vi "Mini Bach random sampling_type2_sub.vi"(0 "Mini Bach No.":i32, 1 "MNIST Input":i32[][](array[numeric])) -> (2 "MNIST Random Output":i32[][](array[numeric]), 3 "MNIST No.Row":i32[](array[numeric]), 4 "MNIST Num":i32[](array[numeric]))   [LabVIEW 2021]
uses:
  <vilib>/numeric/Random Number (Range) I64.vi
  <vilib>/numeric/sub_Random U32.vi
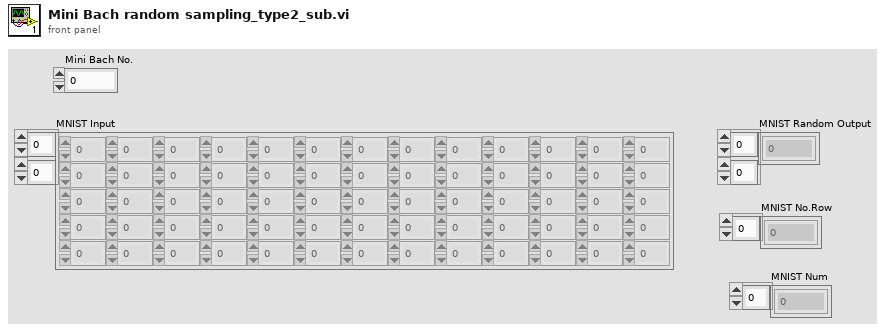
[diagram p1: front panel]
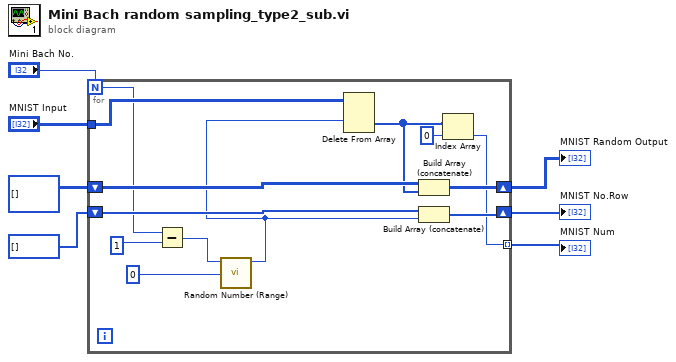
[diagram p0: block diagram]
diagram:
  n1 = for {
    N: "Mini Bach No." -> [w9]
    shift-right: [w20] -> w6
    shift-left: i32[][] [] -> [w19]
    shift-right: [w18] -> w5
    shift-left: i32[] [] -> [w17]
    tunnel: "MNIST Input" -> [w16]
    tunnel: [w11] -> w1 mode=indexing
    n2 = Subtract(x=w9, y=i64 1 ("lower bound (-100)")) -> (x-y=w10:i64)
    n3 = call-poly <vilib>:"Random Number (Range).vi"("lower bound (-100)"=i64 0, "upper bound (100)"=w10) -> ("number"=w14:i64)  [unwired: 9 in]
    n4 = Delete From Array(array=w16, index (row)=w14) -> (deleted portion=w13:i32[])  [unwired: 2 in, 1 out]
    n5 = Build Array (concatenate)(w19, w13) -> (w20:i32[][])
    n6 = Build Array (concatenate)(w17, w14) -> (w18:i64[])
    n7 = Index Array(array=w13, index=0 ("인덱스")) -> (element=w11:i32)
  }
  "MNIST Random Output" <- w6
  "MNIST No.Row" <- w5
  "MNIST Num" <- w1
